vi "Main.vi"() -> ()   [LabVIEW 2024]
doc: "This template is for the Queued Message Handler design pattern.\n\nThe Event Handling Loop generates messages based on user interface actions.\n\nThe Message Handling Loop processes messages generated by the Event Handling Loop, or by other messages. The messages are string values, so new messages can be added easily to the Message Cases case structure in the Message Handling Loop. Each message cluster can also provide an optional value for Message Data, which is a variant that can be converted to whatever message-specific data is required."
uses:
  controls/UI Data.ctl
  <vilib>/Utility/miscctls.llb/LVPointTypeDef.ctl
  <vilib>/Utility/miscctls.llb/LVRectTypeDef.ctl
  support/Message Queue/Enqueue Message (Single).vi
  <vilib>/Instr/_visa.llb/VISA Configure Serial Port (Serial Instr).vi
  support/Message Queue/Message Queue.lvlib
  support/User Event - Stop/User Event - Stop.lvlib
panel:
  in  "Btn-Minimize":bool
  in  "Btn-Close":bool
  in  "Tab ROV":T1(tab)
  in  "Serial-Baudaje":u16(ring) items=["9600"=9600, "19200"=19200, "38400"=38400, "57600"=57600, "115200"=65535]
  in  "Serial-Port":refnum<visa-resource-name>
  in  "Btn-Conectar":bool
  in  "Btn-Desconectar":bool
  out "Serial-State":bool
  out "Numeric 11":dbl
  out "Numeric 10":dbl
  out "Numeric 9":dbl
  out "Numeric 8":dbl
  out "Numeric 7":dbl
  out "Numeric 6":dbl
  out "Numeric 5":dbl
  out "Numeric 4":dbl
  out "Numeric 3":dbl
  out "Numeric 2":dbl
  out "Numeric":dbl
  out "Tecla-S":bool
  out "Tecla-Q":bool
  out "Tecla-E":bool
  out "Tecla-D":bool
  out "Tecla-A":bool
  out "Tecla-W":bool
  in  "Menu4-Propulsores":bool
  in  "Menu3-Inclinacion":bool
  in  "Menu2-Movimientos":bool
  in  "Menu1-Configuracion":bool
  # "Conexión Serial"
  # "Puerto"
  # "Baudaje"
  # "Estado:"
  # "Subir"
  # "Bajar"
  # "Avanzar"
  # "Girar Izquierda"
  # "Retroceder"
  # "Girar Derecha"
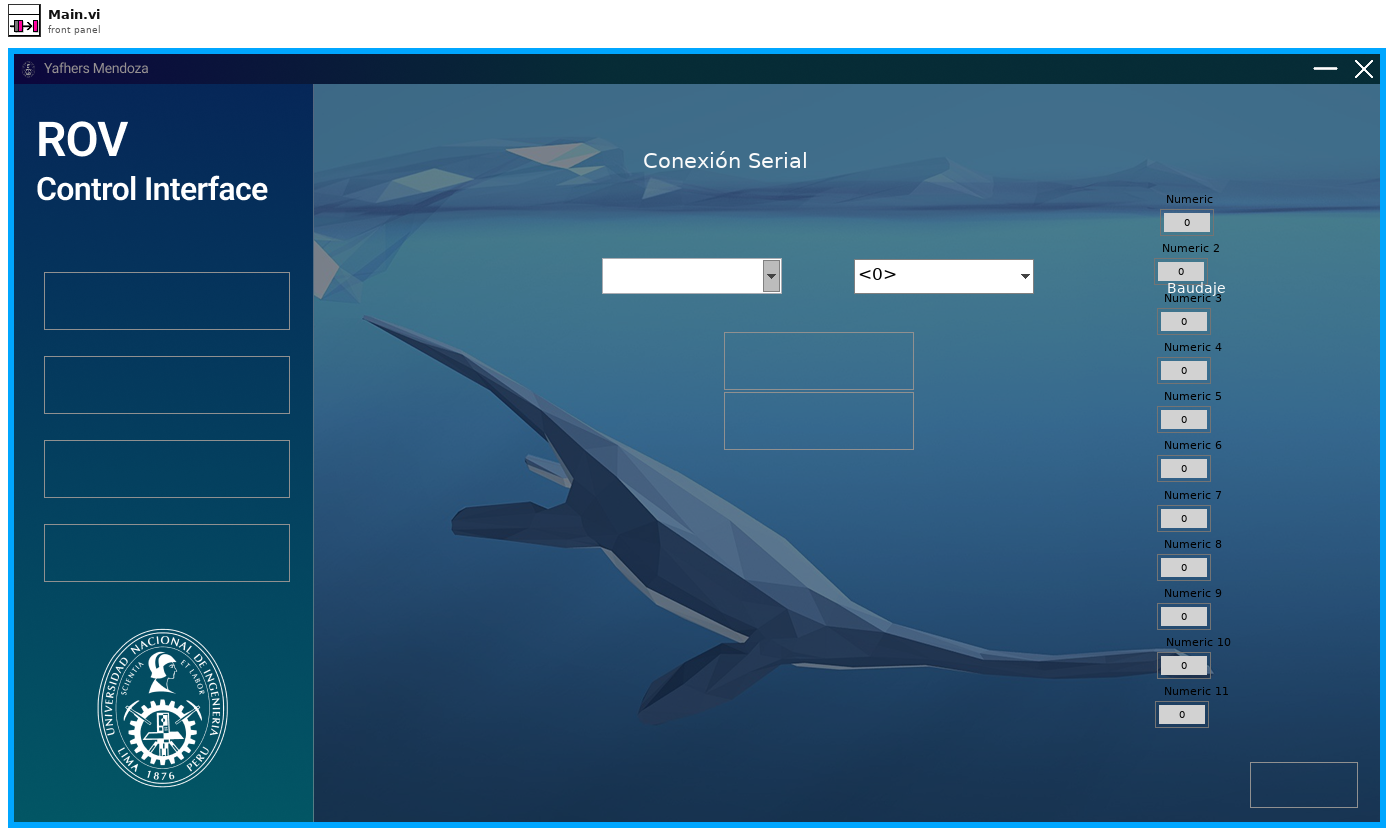
[diagram p1: front panel]
types:
  T1 = enum32{" Tab-Configuracion", "Tab-Movimientos", "Tab-Inclinación", "Tab-Propulsores"}
  T2 = typedef "UI Data.ctl" = cluster{"Data":cluster{"Counter":dbl, "Yaw":dbl, "Pitch":dbl, "Roll":dbl, "Yaw_Desired":dbl, "Pitch_Desired":dbl, "Roll_Desired":dbl, "Motor_Yaw_L":dbl, "Motor_Yaw_R":dbl, "Motor_Pitch_B":dbl, "Motor_Pitch_T":dbl, "Command_Move":dbl}, "Serial":cluster{"Estado":bool, "Puerto":refnum<visa-resource-name>, "Buffer":string}}
  T3 = typedef "Message Queue.lvlib/All Message Queues.ctl" = cluster{"MHL":refnum<queue>, "Loop Serial":refnum<queue>}
  T4 = enum8{"Enabled", "Disabled", "Disabled and Grayed Out"}
  T5 = typedef "LVRectTypeDef.ctl" = cluster{"Left":i16, "Top":i16, "Right":i16, "Bottom":i16}
  T6 = typedef "LVPointTypeDef.ctl" = cluster{"Horizontal":i16, "Vertical":i16}
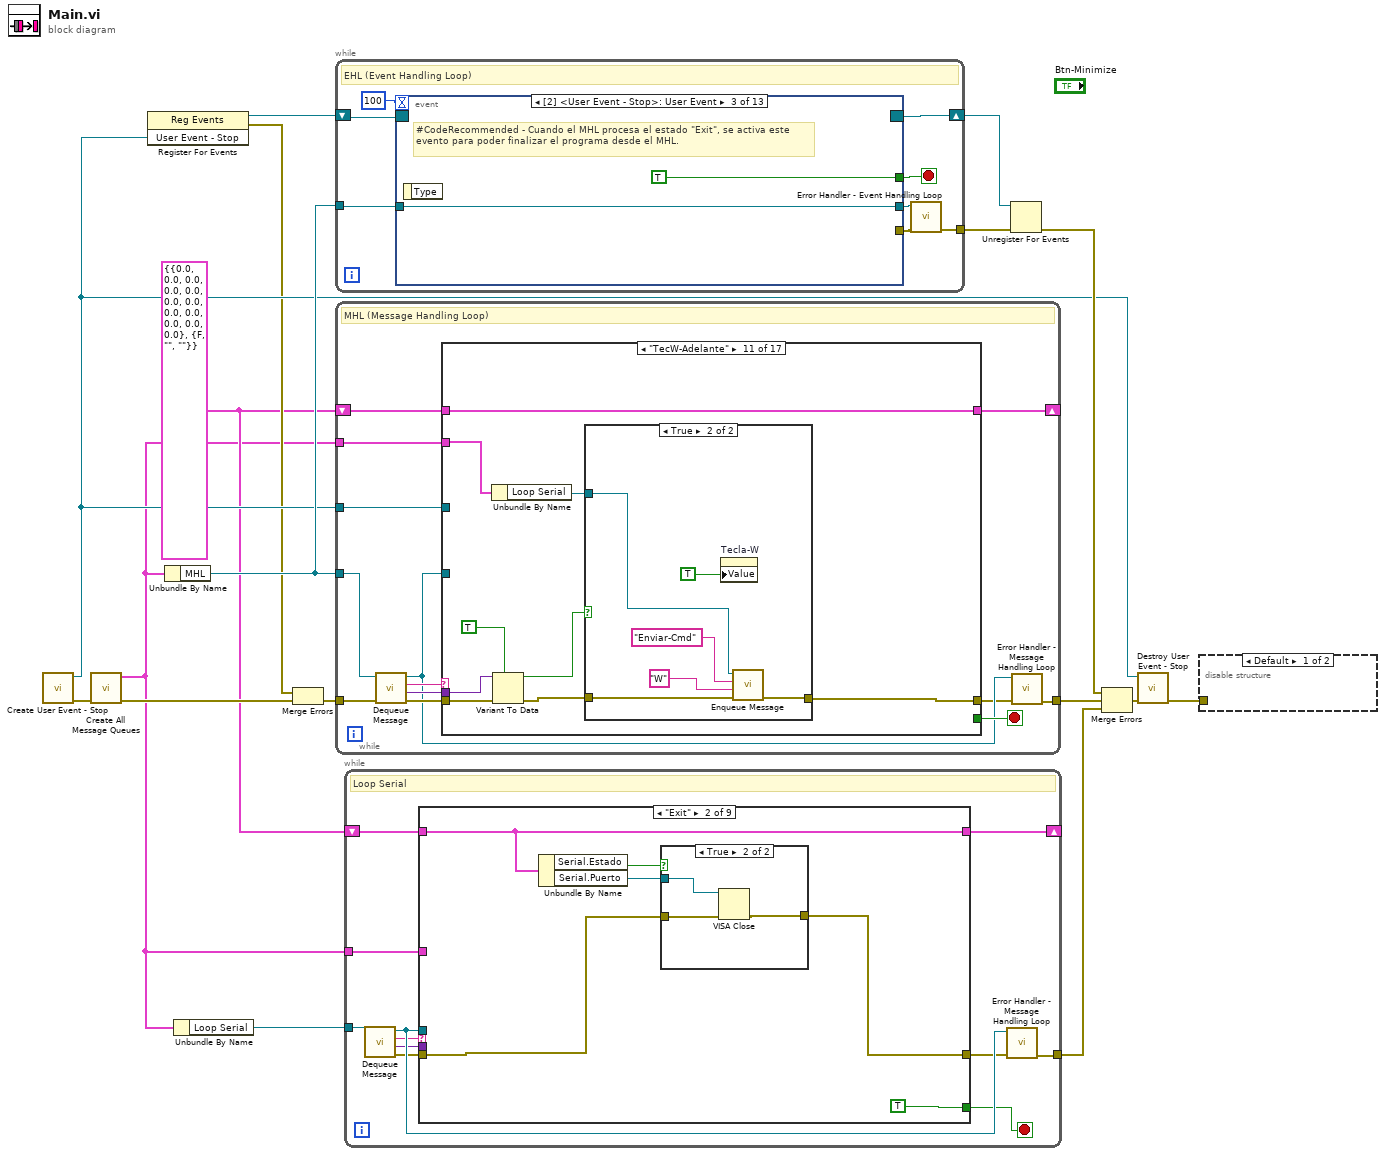
[diagram p0: block diagram]
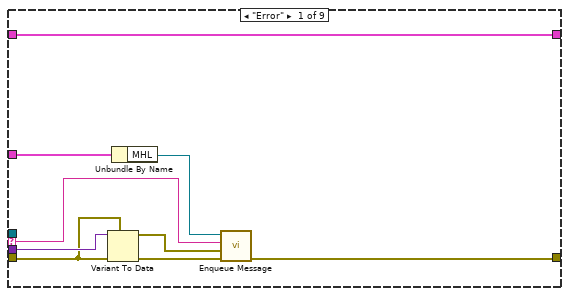
[diagram p2: hidden frame]
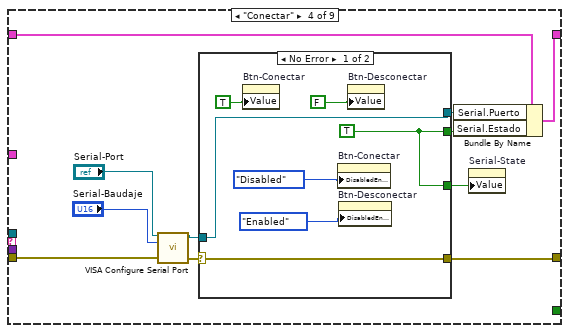
[diagram p5: hidden frame]
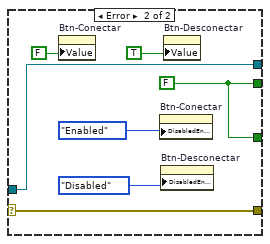
[diagram p6: hidden frame]
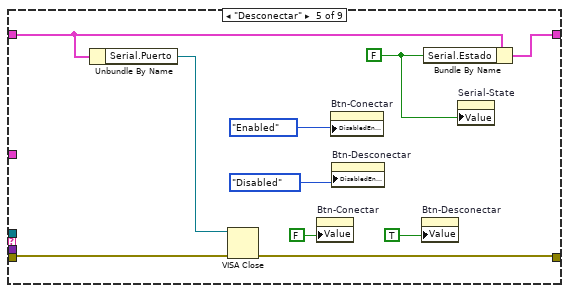
[diagram p7: hidden frame]
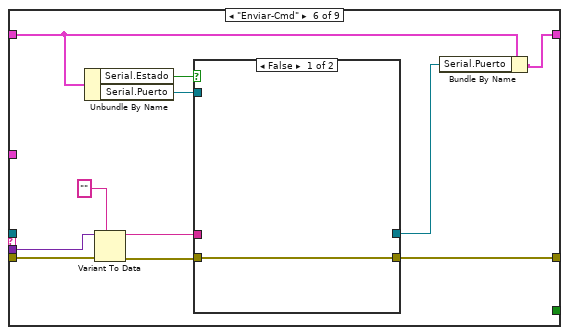
[diagram p8: hidden frame]
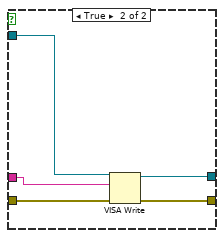
[diagram p9: hidden frame]
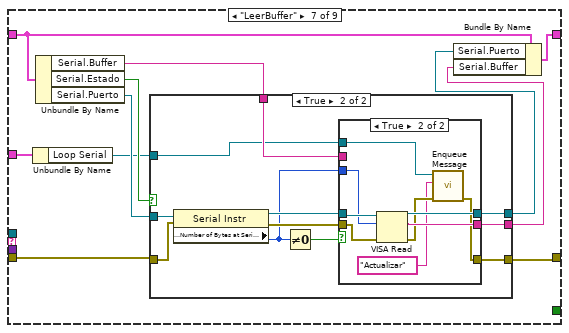
[diagram p10: hidden frame]
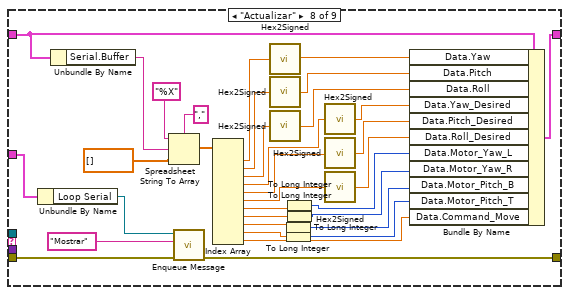
[diagram p13: hidden frame]
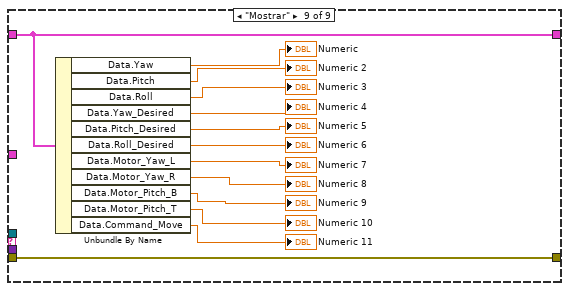
[diagram p14: hidden frame]
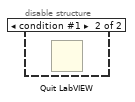
[diagram p15: hidden frame]
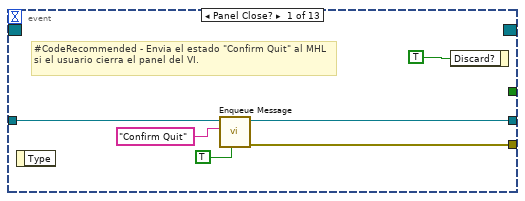
[diagram p16: hidden frame]
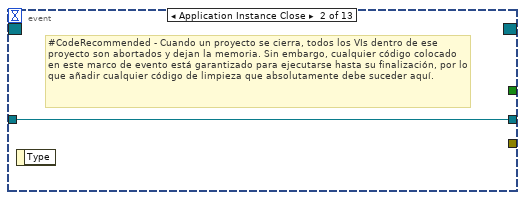
[diagram p17: hidden frame]
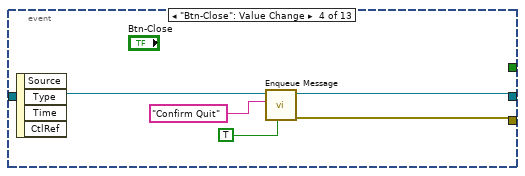
[diagram p18: hidden frame]
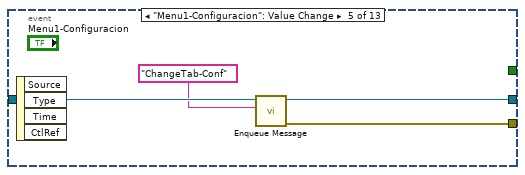
[diagram p19: hidden frame]
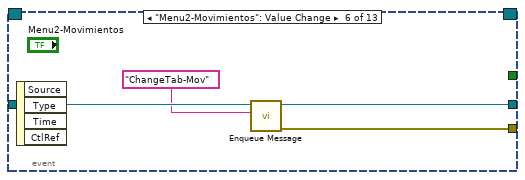
[diagram p20: hidden frame]
diagram:
  w4 = T2 {"Data"={"Counter"=0.0, "Yaw"=0.0, "Pitch"=0.0, "Roll"=0.0, "Yaw_Desired"=0.0, "Pitch_Desired"=0.0, "Roll_Desired"=0.0, "Motor_Yaw_L"=0.0, "Motor_Yaw_R"=0.0, "Motor_Pitch_B"=0.0, "Motor_Pitch_T"=0.0, "Command_Move"=0.0}, "Serial"={"Estado"=FALSE, "Puerto"="", "Buffer"=""}} ("Data Cluster")
  n1 = call "Create User Event - Stop.vi"() -> ("error out"=w14:errorcluster, "User Event - Stop"=w7:refnum<user-event>)  [unwired: 10 in]
  n2 = call "Create All Message Queues.vi"("error in (no error)"=w14) -> ("error out"=w17:errorcluster, "Message Queues out"=w2:T3)  [unwired: 9 in]
  n3 = register-events(w7) -> (reference out=w8:refnum<event-registration>, error out=w5:errorcluster)  [unwired: 2 in]
  n4 = Unbundle By Name(w2) -> ("MHL"=w15:refnum<queue>)
  n5 = Unbundle By Name(w2) -> ("Loop Serial"=w3:refnum<queue>)
  n6 = Merge Errors(w5, w17) -> (w6:errorcluster)
  n7 = while {
    tunnel: w15 -> [w25]
    shift-right: [w23] -> w11
    shift-left: w8 -> [w24]
    tunnel: [w19] -> w9
    stop <- w21 stop-if-true
    # "EHL (Event Handling Loop)"
    n8 = event shown="[2] <User Event - Stop>: User Event" {
      selector: w24 -> [_ _ _ _ _ _ _ _ _ _ _ _ _]
      dyn-events: [_ _ _ _ _ _ _ _ _ _ _ _ _] -> w23
      timeout: 100 -> [_ _ _ _ _ _ _ _ _ _ _ _ _]
      tunnel: [_ _ TRUE ("Discard?") _ _ _ _ _ _ _ _ _ _] -> w21
      tunnel: w25 -> [w30 w32 w34 w37 w43 w47 w51 w55 w59 w63 w67 w102 w137]
      tunnel: [w29 _ _ w38 w42 w46 w50 w54 w58 w61 w66 w101 w135] -> w22
      tunnel: [w28 w32 w34 w39 w41 w45 w49 w53 w57 w62 w65 w100 w136] -> w20
      event Panel Close? {
        # "#CodeRecommended - Envia el estado \"Confirm Quit\" al MHL si el usuario cierra el panel del VI."
        n9 = event-data() -> ()  [unwired: 1 in, 1 out]
        n10 = call-poly "Enqueue Message.vi"("Priority Message? (F)"=TRUE, "Message"="Confirm Quit", "Message Queue"=w30) -> ("error out"=w29:errorcluster, "dup Message Queue"=w28:refnum<queue>)  [unwired: 7 in]
        n11 = event-data("Discard?"=TRUE) -> ()  [unwired: 1 in, 1 out]
      }
      event Application Instance Close {
        # "#CodeRecommended - Cuando un proyecto se cierra, todos los VIs dentro de ese proyecto son abortados y dejan la memoria. Sin embargo, cualquier código colocado en este marco de evento está garantizado para ejecutarse hasta su finalización, por lo que añadir cualquier código de limpieza que absolutamente debe suceder aquí."
        n12 = event-data() -> ()  [unwired: 1 in, 1 out]
      }
      event User Event {
        # "#CodeRecommended - Cuando el MHL procesa el estado \"Exit\", se activa este evento para poder finalizar el programa desde el MHL."
        n13 = event-data() -> ()  [unwired: 1 in, 1 out]
      }
      event "Btn-Close": Value Change {
        n14 = event-data() -> ()  [unwired: 1 in, 4 out]
        n15 = call-poly "Enqueue Message.vi"("Priority Message? (F)"=TRUE, "Message"="Confirm Quit", "Message Queue"=w37) -> ("error out"=w38:errorcluster, "dup Message Queue"=w39:refnum<queue>)  [unwired: 7 in]
      }
      event "Menu1-Configuracion": Value Change {
        n16 = event-data() -> ()  [unwired: 1 in, 4 out]
        n17 = call-poly "Enqueue Message.vi"("Message"="ChangeTab-Conf", "Message Queue"=w43) -> ("error out"=w42:errorcluster, "dup Message Queue"=w41:refnum<queue>)  [unwired: 8 in]
      }
      event "Menu2-Movimientos": Value Change {
        n18 = event-data() -> ()  [unwired: 1 in, 4 out]
        n19 = call-poly "Enqueue Message.vi"("Message"="ChangeTab-Mov", "Message Queue"=w47) -> ("error out"=w46:errorcluster, "dup Message Queue"=w45:refnum<queue>)  [unwired: 8 in]
      }
      event "Menu3-Inclinacion": Value Change {
        n20 = event-data() -> ()  [unwired: 1 in, 4 out]
        n21 = call-poly "Enqueue Message.vi"("Message"="ChangeTab-Inc", "Message Queue"=w51) -> ("error out"=w50:errorcluster, "dup Message Queue"=w49:refnum<queue>)  [unwired: 8 in]
      }
      event "Menu4-Propulsores": Value Change {
        n22 = event-data() -> ()  [unwired: 1 in, 4 out]
        n23 = call-poly "Enqueue Message.vi"("Message"="ChangeTab-Prop", "Message Queue"=w55) -> ("error out"=w54:errorcluster, "dup Message Queue"=w53:refnum<queue>)  [unwired: 8 in]
      }
      event "Btn-Conectar": Value Change {
        n24 = event-data() -> ()  [unwired: 1 in, 4 out]
        n25 = call-poly "Enqueue Message.vi"("Message"="Serial-Conectar", "Message Queue"=w59) -> ("error out"=w58:errorcluster, "dup Message Queue"=w57:refnum<queue>)  [unwired: 8 in]
      }
      event "Btn-Desconectar": Value Change {
        n26 = event-data() -> ()  [unwired: 1 in, 4 out]
        n27 = call-poly "Enqueue Message.vi"("Message"="Serial-Desconectar", "Message Queue"=w63) -> ("error out"=w61:errorcluster, "dup Message Queue"=w62:refnum<queue>)  [unwired: 8 in]
      }
      event Key Down {
        n28 = event-data() -> ("Char"=w64:i16)  [unwired: 1 in, 7 out]
        n29 = case shown="87, 119" w64 {
          tunnel: w67 -> [w68 w73 w78 w83 w88 w93 w98]
          tunnel: [_ w71 w76 w81 w86 w91 w97] -> w66
          tunnel: [w68 w72 w77 w82 w87 w92 w96] -> w65
          frame 0, Default {
          }
          frame 87, 119 {
            # "Tecla W"
            n30 = call-poly "Enqueue Message.vi"("Message Data"=TRUE, "Message"="TecW-Adelante", "Message Queue"=w73) -> ("error out"=w71:errorcluster, "dup Message Queue"=w72:refnum<queue>)  [unwired: 7 in]
          }
          frame 65, 97 {
            # "Tecla A"
            n31 = call-poly "Enqueue Message.vi"("Message Data"=TRUE, "Message"="TecA-GirarIzq", "Message Queue"=w78) -> ("error out"=w76:errorcluster, "dup Message Queue"=w77:refnum<queue>)  [unwired: 7 in]
          }
          frame 68, 100 {
            # "Tecla D"
            n32 = call-poly "Enqueue Message.vi"("Message Data"=TRUE, "Message"="TecD-GirarDer", "Message Queue"=w83) -> ("error out"=w81:errorcluster, "dup Message Queue"=w82:refnum<queue>)  [unwired: 7 in]
          }
          frame 83, 115 {
            # "Tecla S"
            n33 = call-poly "Enqueue Message.vi"("Message Data"=TRUE, "Message"="TecS-Atras", "Message Queue"=w88) -> ("error out"=w86:errorcluster, "dup Message Queue"=w87:refnum<queue>)  [unwired: 7 in]
          }
          frame 81, 113 {
            # "Tecla Q"
            n34 = call-poly "Enqueue Message.vi"("Message Data"=TRUE, "Message"="TecQ-Bajar", "Message Queue"=w93) -> ("error out"=w91:errorcluster, "dup Message Queue"=w92:refnum<queue>)  [unwired: 7 in]
          }
          frame 69, 101 {
            # "Tecla E"
            n35 = call-poly "Enqueue Message.vi"("Message Data"=TRUE, "Message"="TecE-Subir", "Message Queue"=w98) -> ("error out"=w97:errorcluster, "dup Message Queue"=w96:refnum<queue>)  [unwired: 7 in]
          }
        }
      }
      event Key Up {
        n36 = event-data() -> ("ScanCode"=w99:i16)  [unwired: 1 in, 7 out]
        n37 = case shown="0, Default" w99 {
          tunnel: w102 -> [w103 w108 w113 w118 w123 w128 w133]
          tunnel: [_ w106 w111 w116 w121 w126 w132] -> w101
          tunnel: [w103 w107 w112 w117 w122 w127 w131] -> w100
          frame 0, Default {
          }
          frame 17 {
            # "Tecla W"
            n38 = call-poly "Enqueue Message.vi"("Message Data"=FALSE, "Message"="TecW-Adelante", "Message Queue"=w108) -> ("error out"=w106:errorcluster, "dup Message Queue"=w107:refnum<queue>)  [unwired: 7 in]
          }
          frame 30 {
            # "Tecla A"
            n39 = call-poly "Enqueue Message.vi"("Message Data"=FALSE, "Message"="TecA-GirarIzq", "Message Queue"=w113) -> ("error out"=w111:errorcluster, "dup Message Queue"=w112:refnum<queue>)  [unwired: 7 in]
          }
          frame 32 {
            # "Tecla D"
            n40 = call-poly "Enqueue Message.vi"("Message Data"=FALSE, "Message"="TecD-GirarDer", "Message Queue"=w118) -> ("error out"=w116:errorcluster, "dup Message Queue"=w117:refnum<queue>)  [unwired: 7 in]
          }
          frame 31 {
            # "Tecla S"
            n41 = call-poly "Enqueue Message.vi"("Message Data"=FALSE, "Message"="TecS-Atras", "Message Queue"=w123) -> ("error out"=w121:errorcluster, "dup Message Queue"=w122:refnum<queue>)  [unwired: 7 in]
          }
          frame 16 {
            # "Tecla Q"
            n42 = call-poly "Enqueue Message.vi"("Message Data"=FALSE, "Message"="TecQ-Bajar", "Message Queue"=w128) -> ("error out"=w126:errorcluster, "dup Message Queue"=w127:refnum<queue>)  [unwired: 7 in]
          }
          frame 18 {
            # "Tecla E"
            n43 = call-poly "Enqueue Message.vi"("Message Data"=FALSE, "Message"="TecE-Subir", "Message Queue"=w133) -> ("error out"=w132:errorcluster, "dup Message Queue"=w131:refnum<queue>)  [unwired: 7 in]
          }
        }
      }
      event Timeout {
        n44 = event-data() -> ()  [unwired: 1 in, 3 out]
        n45 = call-poly "Enqueue Message.vi"("Message"="Serial-CollectData", "Message Queue"=w137) -> ("error out"=w135:errorcluster, "dup Message Queue"=w136:refnum<queue>)  [unwired: 8 in]
      }
    }
    n46 = call "Error Handler - Event Handling Loop.vi"("error in (no error)"=w22, "Message Queue"=w20) -> ("dup error in"=w19:errorcluster)  [unwired: 8 in, 1 out]
  }
  n47 = while {
    tunnel: w15 -> [w142]
    shift-right: [w149] -> _
    shift-left: w4 -> [w150]
    tunnel: w7 -> [w147]
    tunnel: w6 -> [w146]
    tunnel: [w140] -> w16
    tunnel: w2 -> [w138]
    stop <- w148 stop-if-true
    # "MHL (Message Handling Loop)"
    n48 = call "Dequeue Message.vi"("error in (no error)"=w146, "Message Queue"=w142) -> ("error out"=w145:errorcluster, "Message Data"=w143:variant, "Message"=w144:string, "dup Message Queue"=w141:refnum<queue>)  [unwired: 6 in]
    n49 = case "Message Cases" shown="\"TecW-Adelante\"" w144 {
      tunnel: w141 -> [_ _ w189 _ _ _ _ _ _ _ _ _ _ _ _ _ w375]
      tunnel: w145 -> [w173 w180 w192 w199 w206 w213 w220 w224 w230 w236 w246 w266 w287 w308 w329 w350 w368]
      tunnel: [w173 w174 w190 w199 w206 w213 w220 w223 w227 w235 w240 w262 w282 w304 w325 w346 w371] -> w139
      tunnel: w150 -> [w172 w179 w191 w198 w205 w212 w219 w226 w232 w238 w247 w268 w289 w310 w331 w352 w374]
      tunnel: [w172 w179 w191 w198 w205 w212 w219 w226 w232 w238 w247 w268 w289 w310 w331 w352 w374] -> w149
      tunnel: [_ _ _ _ _ _ _ _ _ _ _ _ _ _ _ _ TRUE] -> w148
      tunnel: w143 -> [_ w178 _ _ _ _ _ _ _ _ w245 w265 w286 w306 w328 w349 w365]
      tunnel: w147 -> [_ _ _ _ _ _ _ _ _ _ _ _ _ _ _ _ w370]
      tunnel: w138 -> [_ _ w186 _ _ _ _ w225 w231 w237 w242 w261 w284 w303 w324 w345 _]
      frame "Initialize", Default {
        w153 = FALSE ("Serial-State")
        # "#CodeRecommended - Estado de Inicialización por defecto."
        # "Initialize - All initialization work should take place in this message, since other loops can potentially enqueue messages that execute immediately after this one."
        n50 = property on="Pane" class="Pane"("Origin"=T6 {"Horizontal"=0, "Vertical"=0}) -> ()  [unwired: 2 in, 2 out]
        n51 = Current VI's Path() -> (path=w169:path)
        n52 = property on="Btn-Conectar" class="Bool (strict)"("DisabledEnum"=T4."Enabled" ("Disabled")) -> ()  [unwired: 2 in, 2 out]
        n53 = property on="Menu3-Inclinacion" class="Bool (strict)"("DisabledEnum"=T4."Disabled" ("Disabled")) -> ()  [unwired: 2 in, 2 out]
        n54 = property on="Menu4-Propulsores" class="Bool (strict)"("DisabledEnum"=T4."Disabled" ("Disabled")) -> ()  [unwired: 2 in, 2 out]
        n55 = property on="Btn-Desconectar" class="Bool (strict)"("DisabledEnum"=T4."Enabled" ("Disabled")) -> ()  [unwired: 2 in, 2 out]
        n56 = Open VI Reference(vi path=w169) -> (vi reference=w168:refnum<vi>, error out=w167:errorcluster)  [unwired: 5 in]
        n57 = property on="Tab ROV" class="TabCtl (strict)"("Value"=T1." Tab-Configuracion" ("Tab ROV")) -> ()  [unwired: 2 in, 2 out]
        n58 = property class="VI"(reference=w168, error in=w167, "Front Panel.PanelBounds"=T5 {"Left"=300, "Top"=120, "Right"=1366, "Bottom"=768} ("Front Panel Window:Panel Bounds")) -> (reference out=w166:refnum<vi>, error out=w165:errorcluster)
        n59 = property on="Menu4-Propulsores" class="Bool (strict)"("Value"=FALSE) -> ()  [unwired: 2 in, 2 out]
        n60 = property on="Menu2-Movimientos" class="Bool (strict)"("Value"=FALSE) -> ()  [unwired: 2 in, 2 out]
        n61 = property on="Menu1-Configuracion" class="Bool (strict)"("Value"=TRUE) -> ()  [unwired: 2 in, 2 out]
        n62 = property on="Menu3-Inclinacion" class="Bool (strict)"("Value"=FALSE) -> ()  [unwired: 2 in, 2 out]
        n63 = property on="Btn-Conectar" class="Bool (strict)"("Value"=FALSE) -> ()  [unwired: 2 in, 2 out]
        n64 = Close Reference(reference=w166, error in (no error)=w165) -> ()  [unwired: 1 out]
        n65 = property on="Btn-Desconectar" class="Bool (strict)"("Value"=FALSE) -> ()  [unwired: 2 in, 2 out]
        n66 = property on="Serial-State" class="Bool"("Value"=FALSE) -> ()  [unwired: 2 in, 2 out]
        "Serial-State" <- FALSE ("Serial-State")
        "Tecla-W" <- w153
        "Tecla-D" <- w153
        "Tecla-A" <- w153
        "Tecla-S" <- w153
        "Tecla-Q" <- w153
        "Tecla-E" <- w153
      }
      frame "Error" {
        # "#CodeRecommended - Muestra un diálogo de error. Este mensaje es enviado por los VIs «Error Handler» al final de otros bucles en esta aplicación.."
        # "Error - Display an error dialog. This message is sent by the \"Error Handler\" VIs at the end of other loops in this application."
        n67 = Variant To Data(error in=w180, type=errorcluster {"status"=FALSE, "code"=0, "source"=""} ("error constant"), Variant=w178) -> (data=w176:errorcluster, error out=w175:errorcluster)
        n68 = call <vilib>:"Simple Error Handler.vi"("error in (no error)"=w176) -> ()  [unwired: 4 in, 5 out]
        n69 = Merge Errors(w175) -> (w174:errorcluster)
      }
      frame "Confirm Quit" {
        # "#CodeRecommended - Estado para confirmar que el usuario desea salir de la aplicación, asegurese de cerrar todos sus bucles en este estado."
        # "Confirm Quit - Message that can confirm whether or not the user wants to exit the application."
        n70 = Unbundle By Name(w186) -> ("Loop Serial"=w184:refnum<queue>)
        n71 = call-poly "Enqueue Message.vi"("Priority Message? (F)"=TRUE, "error in (no error)"=w192, "Message"="Exit", "Message Queue"=w189) -> ("error out"=w185:errorcluster)  [unwired: 6 in, 1 out]
        n72 = call-poly "Enqueue Message.vi"("Priority Message? (F)"=TRUE, "error in (no error)"=w185, "Message"="Exit", "Message Queue"=w184) -> ("error out"=w181:errorcluster)  [unwired: 6 in, 1 out]
        n73 = Merge Errors(w181) -> (w190:errorcluster)
      }
      frame "ChangeTab-Conf" {
        n74 = property on="Menu2-Movimientos" class="Bool (strict)"("Value"=FALSE) -> ()  [unwired: 2 in, 2 out]
        n75 = property on="Menu1-Configuracion" class="Bool (strict)"("Value"=TRUE) -> ()  [unwired: 2 in, 2 out]
        n76 = property on="Menu4-Propulsores" class="Bool (strict)"("Value"=FALSE) -> ()  [unwired: 2 in, 2 out]
        n77 = property on="Menu3-Inclinacion" class="Bool (strict)"("Value"=FALSE) -> ()  [unwired: 2 in, 2 out]
        n78 = property on="Tab ROV" class="TabCtl (strict)"("Value"=T1." Tab-Configuracion" ("Tab ROV")) -> ()  [unwired: 2 in, 2 out]
      }
      frame "ChangeTab-Mov" {
        n79 = property on="Menu2-Movimientos" class="Bool (strict)"("Value"=TRUE) -> ()  [unwired: 2 in, 2 out]
        n80 = property on="Menu1-Configuracion" class="Bool (strict)"("Value"=FALSE) -> ()  [unwired: 2 in, 2 out]
        n81 = property on="Menu4-Propulsores" class="Bool (strict)"("Value"=FALSE) -> ()  [unwired: 2 in, 2 out]
        n82 = property on="Menu3-Inclinacion" class="Bool (strict)"("Value"=FALSE) -> ()  [unwired: 2 in, 2 out]
        n83 = property on="Tab ROV" class="TabCtl (strict)"("Value"=T1."Tab-Movimientos" ("Tab ROV")) -> ()  [unwired: 2 in, 2 out]
      }
      frame "ChangeTab-Inc" {
        n84 = property on="Menu2-Movimientos" class="Bool (strict)"("Value"=FALSE) -> ()  [unwired: 2 in, 2 out]
        n85 = property on="Menu1-Configuracion" class="Bool (strict)"("Value"=FALSE) -> ()  [unwired: 2 in, 2 out]
        n86 = property on="Menu4-Propulsores" class="Bool (strict)"("Value"=FALSE) -> ()  [unwired: 2 in, 2 out]
        n87 = property on="Menu3-Inclinacion" class="Bool (strict)"("Value"=TRUE) -> ()  [unwired: 2 in, 2 out]
        n88 = property on="Tab ROV" class="TabCtl (strict)"("Value"=T1."Tab-Inclinación" ("Tab ROV")) -> ()  [unwired: 2 in, 2 out]
      }
      frame "ChangeTab-Prop" {
        n89 = property on="Menu2-Movimientos" class="Bool (strict)"("Value"=FALSE) -> ()  [unwired: 2 in, 2 out]
        n90 = property on="Menu1-Configuracion" class="Bool (strict)"("Value"=FALSE) -> ()  [unwired: 2 in, 2 out]
        n91 = property on="Menu4-Propulsores" class="Bool (strict)"("Value"=TRUE) -> ()  [unwired: 2 in, 2 out]
        n92 = property on="Menu3-Inclinacion" class="Bool (strict)"("Value"=FALSE) -> ()  [unwired: 2 in, 2 out]
        n93 = property on="Tab ROV" class="TabCtl (strict)"("Value"=T1."Tab-Propulsores" ("Tab ROV")) -> ()  [unwired: 2 in, 2 out]
      }
      frame "Serial-Conectar" {
        n94 = Unbundle By Name(w225) -> ("Loop Serial"=w222:refnum<queue>)
        n95 = call-poly "Enqueue Message.vi"("error in (no error)"=w224, "Message"="Conectar", "Message Queue"=w222) -> ("error out"=w223:errorcluster)  [unwired: 7 in, 1 out]
      }
      frame "Serial-Desconectar" {
        n96 = Unbundle By Name(w231) -> ("Loop Serial"=w229:refnum<queue>)
        n97 = call-poly "Enqueue Message.vi"("error in (no error)"=w230, "Message"="Desconectar", "Message Queue"=w229) -> ("error out"=w227:errorcluster)  [unwired: 7 in, 1 out]
      }
      frame "Serial-CollectData" {
        n98 = Unbundle By Name(w237) -> ("Loop Serial"=w234:refnum<queue>)
        n99 = call-poly "Enqueue Message.vi"("error in (no error)"=w236, "Message"="LeerBuffer", "Message Queue"=w234) -> ("error out"=w235:errorcluster)  [unwired: 7 in, 1 out]
      }
      frame "TecW-Adelante" {
        n100 = Unbundle By Name(w242) -> ("Loop Serial"=w239:refnum<queue>)
        n101 = Variant To Data(error in=w246, type=TRUE, Variant=w245) -> (data=w243:bool, error out=w241:errorcluster)
        n102 = case shown="True" w243 {
          tunnel: w241 -> [w252 w256]
          tunnel: [w251 w255] -> w240
          tunnel: w239 -> [w249 w254]
          frame False {
            n103 = property on="Tecla-W" class="Bool"("Value"=FALSE ("Tecla-W")) -> ()  [unwired: 2 in, 2 out]
            n104 = call-poly "Enqueue Message.vi"("error in (no error)"=w252, "Message Data"="w", "Message"="Enviar-Cmd", "Message Queue"=w249) -> ("error out"=w251:errorcluster)  [unwired: 6 in, 1 out]
          }
          frame True {
            n105 = property on="Tecla-W" class="Bool"("Value"=TRUE ("Tecla-W")) -> ()  [unwired: 2 in, 2 out]
            n106 = call-poly "Enqueue Message.vi"("error in (no error)"=w256, "Message Data"="W", "Message"="Enviar-Cmd", "Message Queue"=w254) -> ("error out"=w255:errorcluster)  [unwired: 6 in, 1 out]
          }
        }
      }
      frame "TecD-GirarDer" {
        n107 = Unbundle By Name(w261) -> ("Loop Serial"=w260:refnum<queue>)
        n108 = Variant To Data(error in=w266, type=TRUE, Variant=w265) -> (data=w264:bool, error out=w263:errorcluster)
        n109 = case shown="True" w264 {
          tunnel: w263 -> [w271 w277]
          tunnel: [w270 w276] -> w262
          tunnel: w260 -> [w269 w275]
          frame False {
            n110 = property on="Tecla-D" class="Bool"("Value"=FALSE ("Tecla-D")) -> ()  [unwired: 2 in, 2 out]
            n111 = call-poly "Enqueue Message.vi"("error in (no error)"=w271, "Message Data"="d", "Message"="Enviar-Cmd", "Message Queue"=w269) -> ("error out"=w270:errorcluster)  [unwired: 6 in, 1 out]
          }
          frame True {
            n112 = property on="Tecla-D" class="Bool"("Value"=TRUE ("Tecla-D")) -> ()  [unwired: 2 in, 2 out]
            n113 = call-poly "Enqueue Message.vi"("error in (no error)"=w277, "Message Data"="D", "Message"="Enviar-Cmd", "Message Queue"=w275) -> ("error out"=w276:errorcluster)  [unwired: 6 in, 1 out]
          }
        }
      }
      frame "TecA-GirarIzq" {
        n114 = Unbundle By Name(w284) -> ("Loop Serial"=w281:refnum<queue>)
        n115 = Variant To Data(error in=w287, type=TRUE, Variant=w286) -> (data=w285:bool, error out=w283:errorcluster)
        n116 = case shown="True" w285 {
          tunnel: w283 -> [w292 w298]
          tunnel: [w291 w297] -> w282
          tunnel: w281 -> [w290 w296]
          frame False {
            n117 = property on="Tecla-A" class="Bool"("Value"=FALSE ("Tecla-A")) -> ()  [unwired: 2 in, 2 out]
            n118 = call-poly "Enqueue Message.vi"("error in (no error)"=w292, "Message Data"="a", "Message"="Enviar-Cmd", "Message Queue"=w290) -> ("error out"=w291:errorcluster)  [unwired: 6 in, 1 out]
          }
          frame True {
            n119 = property on="Tecla-A" class="Bool"("Value"=TRUE ("Tecla-A")) -> ()  [unwired: 2 in, 2 out]
            n120 = call-poly "Enqueue Message.vi"("error in (no error)"=w298, "Message Data"="A", "Message"="Enviar-Cmd", "Message Queue"=w296) -> ("error out"=w297:errorcluster)  [unwired: 6 in, 1 out]
          }
        }
      }
      frame "TecS-Atras" {
        n121 = Unbundle By Name(w303) -> ("Loop Serial"=w302:refnum<queue>)
        n122 = Variant To Data(error in=w308, type=TRUE, Variant=w306) -> (data=w307:bool, error out=w305:errorcluster)
        n123 = case shown="False" w307 {
          tunnel: w305 -> [w313 w319]
          tunnel: [w312 w318] -> w304
          tunnel: w302 -> [w311 w317]
          frame False {
            n124 = property on="Tecla-S" class="Bool"("Value"=FALSE ("Tecla-S")) -> ()  [unwired: 2 in, 2 out]
            n125 = call-poly "Enqueue Message.vi"("error in (no error)"=w313, "Message Data"="s", "Message"="Enviar-Cmd", "Message Queue"=w311) -> ("error out"=w312:errorcluster)  [unwired: 6 in, 1 out]
          }
          frame True {
            n126 = property on="Tecla-S" class="Bool"("Value"=TRUE ("Tecla-S")) -> ()  [unwired: 2 in, 2 out]
            n127 = call-poly "Enqueue Message.vi"("error in (no error)"=w319, "Message Data"="S", "Message"="Enviar-Cmd", "Message Queue"=w317) -> ("error out"=w318:errorcluster)  [unwired: 6 in, 1 out]
          }
        }
      }
      frame "TecQ-Bajar" {
        n128 = Unbundle By Name(w324) -> ("Loop Serial"=w323:refnum<queue>)
        n129 = Variant To Data(error in=w329, type=TRUE, Variant=w328) -> (data=w327:bool, error out=w326:errorcluster)
        n130 = case shown="False" w327 {
          tunnel: w326 -> [w334 w340]
          tunnel: [w333 w339] -> w325
          tunnel: w323 -> [w332 w338]
          frame False {
            n131 = property on="Tecla-Q" class="Bool"("Value"=FALSE ("Tecla-Q")) -> ()  [unwired: 2 in, 2 out]
            n132 = call-poly "Enqueue Message.vi"("error in (no error)"=w334, "Message Data"="q", "Message"="Enviar-Cmd", "Message Queue"=w332) -> ("error out"=w333:errorcluster)  [unwired: 6 in, 1 out]
          }
          frame True {
            n133 = property on="Tecla-Q" class="Bool"("Value"=TRUE ("Tecla-Q")) -> ()  [unwired: 2 in, 2 out]
            n134 = call-poly "Enqueue Message.vi"("error in (no error)"=w340, "Message Data"="Q", "Message"="Enviar-Cmd", "Message Queue"=w338) -> ("error out"=w339:errorcluster)  [unwired: 6 in, 1 out]
          }
        }
      }
      frame "TecE-Subir" {
        n135 = Unbundle By Name(w345) -> ("Loop Serial"=w344:refnum<queue>)
        n136 = Variant To Data(error in=w350, type=TRUE, Variant=w349) -> (data=w348:bool, error out=w347:errorcluster)
        n137 = case shown="False" w348 {
          tunnel: w347 -> [w355 w361]
          tunnel: [w354 w360] -> w346
          tunnel: w344 -> [w353 w359]
          frame False {
            n138 = property on="Tecla-E" class="Bool"("Value"=FALSE ("Tecla-E")) -> ()  [unwired: 2 in, 2 out]
            n139 = call-poly "Enqueue Message.vi"("error in (no error)"=w355, "Message Data"="e", "Message"="Enviar-Cmd", "Message Queue"=w353) -> ("error out"=w354:errorcluster)  [unwired: 6 in, 1 out]
          }
          frame True {
            n140 = property on="Tecla-E" class="Bool"("Value"=TRUE ("Tecla-E")) -> ()  [unwired: 2 in, 2 out]
            n141 = call-poly "Enqueue Message.vi"("error in (no error)"=w361, "Message Data"="E", "Message"="Enviar-Cmd", "Message Queue"=w359) -> ("error out"=w360:errorcluster)  [unwired: 6 in, 1 out]
          }
        }
      }
      frame "Exit" {
        # "#CodeRecommended - Añada aquí cualquier código de limpieza necesario. Tenga en cuenta que si 'EXIT' fue llamado como resultado de un error, se mostrará un diálogo de error. Añada también aquí cualquier gestión de error personalizada para una condición 'Salir'."
        # "Exit - Exit the application."
        n142 = Variant To Data(type=errorcluster {"status"=FALSE, "code"=0, "source"=""} ("error constant"), Variant=w365) -> (data=w366:errorcluster)  [unwired: 1 in, 1 out]
        n143 = call <vilib>:"Simple Error Handler.vi"("error in (no error)"=w366) -> ()  [unwired: 4 in, 5 out]
        n144 = call "Fire User Event - Stop.vi"("User Event - Stop"=w370) -> ("error out"=w369:errorcluster)  [unwired: 10 in]
        n145 = Release Queue(queue=w375, error in (no error)=w368) -> (error out=w372:errorcluster)  [unwired: 1 in, 2 out]
        n146 = Merge Errors(w369, w372) -> (w371:errorcluster)
      }
    }
    n147 = call "Error Handler - Message Handling Loop.vi"("error in (no error)"=w139, "Message Queue"=w141) -> ("dup error in"=w140:errorcluster)  [unwired: 8 in, 1 out]
  }
  n148 = while {
    shift-right: [w379] -> _
    shift-left: w4 -> [w378]
    tunnel: [w381] -> w1
    tunnel: w3 -> [w380]
    tunnel: w2 -> [w377]
    stop <- w376 stop-if-true
    # "Loop Serial"
    n149 = call "Dequeue Message.vi"("Message Queue"=w380) -> ("error out"=w384:errorcluster, "Message Data"=w383:variant, "Message"=w385:string, "dup Message Queue"=w386:refnum<queue>)  [unwired: 7 in]
    n150 = case shown="\"Exit\"" w385 {
      selector: w385 -> [w389 _ _ _ _ _ _ _ _]
      tunnel: w386 -> [_ _ _ _ _ _ _ _ _]
      tunnel: w384 -> [w393 w397 w407 w418 w442 w447 w468 w521 w541]
      tunnel: w383 -> [w394 _ _ _ _ w445 _ _ _]
      tunnel: [w387 w396 w407 w411 w440 w452 w469 w520 w541] -> w382
      tunnel: [w395 w400 w406 w414 w438 w449 w465 w529 w542] -> w379
      tunnel: w378 -> [w395 w400 w406 w413 w439 w450 w466 w528 w542]
      tunnel: w377 -> [w392 _ _ _ _ _ w461 w519 _]
      tunnel: [_ TRUE _ _ _ _ _ _ _] -> w376
      frame "Error" {
        n151 = Variant To Data(error in=w393, type=w393, Variant=w394) -> (data=w388:errorcluster, error out=w391:errorcluster)
        n152 = Unbundle By Name(w392) -> ("MHL"=w390:refnum<queue>)
        n153 = call-poly "Enqueue Message.vi"("error in (no error)"=w391, "Message Data"=w388, "Message"=w389, "Message Queue"=w390) -> ("error out"=w387:errorcluster)  [unwired: 6 in, 1 out]
      }
      frame "Exit" {
        n154 = Unbundle By Name(w400) -> ("Serial.Estado"=w399:bool, "Serial.Puerto"=w398:refnum<visa-resource-name>)
        n155 = case shown="True" w399 {
          tunnel: w398 -> [_ w405]
          tunnel: w397 -> [w402 w404]
          tunnel: [w402 w403] -> w396
          frame False {
          }
          frame True {
            n156 = VISA Close(VISA resource name=w405, error in (no error)=w404) -> (error out=w403:errorcluster)
          }
        }
      }
      frame "Initialize", Default {
      }
      frame "Conectar" {
        n157 = call-poly "VISA Configure Serial Port"("VISA resource name"="Serial-Port", "baud rate (9600)"="Serial-Baudaje", "error in (no error)"=w418) -> ("VISA resource name out"=w412:refnum<visa-resource-name>, "error out"=w415:errorcluster)  [unwired: 11 in]
        n158 = case shown="No Error" w415 {
          selector: w415 -> [w424 w431]
          tunnel: [w425 w432] -> w410
          tunnel: w412 -> [w425 w432]
          tunnel: [w424 w431] -> w411
          tunnel: [w421 w428] -> w409
          tunnel: [w421 w428] -> w408
          frame No Error {
            w421 = TRUE
            n159 = property on="Btn-Conectar" class="Bool (strict)"("Value"=TRUE ("Btn-Conectar")) -> ()  [unwired: 2 in, 2 out]
            n160 = property on="Btn-Conectar" class="Bool (strict)"("DisabledEnum"=T4."Disabled" ("Disabled")) -> ()  [unwired: 2 in, 2 out]
            n161 = property on="Btn-Desconectar" class="Bool (strict)"("DisabledEnum"=T4."Enabled" ("Disabled")) -> ()  [unwired: 2 in, 2 out]
            n162 = property on="Btn-Desconectar" class="Bool (strict)"("Value"=FALSE ("Btn-Desconectar")) -> ()  [unwired: 2 in, 2 out]
          }
          frame Error {
            w428 = FALSE
            n163 = property on="Btn-Conectar" class="Bool (strict)"("Value"=FALSE ("Btn-Conectar")) -> ()  [unwired: 2 in, 2 out]
            n164 = property on="Btn-Conectar" class="Bool (strict)"("DisabledEnum"=T4."Enabled" ("Disabled")) -> ()  [unwired: 2 in, 2 out]
            n165 = property on="Btn-Desconectar" class="Bool (strict)"("DisabledEnum"=T4."Disabled" ("Disabled")) -> ()  [unwired: 2 in, 2 out]
            n166 = property on="Btn-Desconectar" class="Bool (strict)"("Value"=TRUE ("Btn-Desconectar")) -> ()  [unwired: 2 in, 2 out]
          }
        }
        n167 = Bundle By Name(cluster=w413, "Serial.Puerto"=w410, "Serial.Estado"=w409) -> (w414:T2)
        n168 = property on="Serial-State" class="Bool"("Value"=w408) -> ()  [unwired: 2 in, 2 out]
      }
      frame "Desconectar" {
        w437 = FALSE ("Serial.Estado")
        n169 = Unbundle By Name(w439) -> ("Serial.Puerto"=w441:refnum<visa-resource-name>)
        n170 = VISA Close(VISA resource name=w441, error in (no error)=w442) -> (error out=w440:errorcluster)
        n171 = property on="Btn-Conectar" class="Bool (strict)"("Value"=FALSE ("Btn-Conectar")) -> ()  [unwired: 2 in, 2 out]
        n172 = property on="Btn-Conectar" class="Bool (strict)"("DisabledEnum"=T4."Enabled" ("Disabled")) -> ()  [unwired: 2 in, 2 out]
        n173 = property on="Btn-Desconectar" class="Bool (strict)"("DisabledEnum"=T4."Disabled" ("Disabled")) -> ()  [unwired: 2 in, 2 out]
        n174 = property on="Btn-Desconectar" class="Bool (strict)"("Value"=TRUE ("Btn-Desconectar")) -> ()  [unwired: 2 in, 2 out]
        n175 = Bundle By Name(cluster=w439, "Serial.Estado"=w437) -> (w438:T2)
        n176 = property on="Serial-State" class="Bool"("Value"=w437) -> ()  [unwired: 2 in, 2 out]
      }
      frame "Enviar-Cmd" {
        n177 = Unbundle By Name(w450) -> ("Serial.Estado"=w453:bool, "Serial.Puerto"=w451:refnum<visa-resource-name>)
        n178 = Variant To Data(error in=w447, type="", Variant=w445) -> (data=w443:string, error out=w446:errorcluster)
        n179 = case shown="False" w453 {
          tunnel: w446 -> [w454 w459]
          tunnel: [w454 w458] -> w452
          tunnel: w451 -> [_ w457]
          tunnel: [_ w456] -> w448
          tunnel: w443 -> [_ w455]
          frame False {
          }
          frame True {
            n180 = VISA Write(VISA resource name=w457, write buffer=w455, error in (no error)=w459) -> (VISA resource name out=w456:refnum<visa-resource-name>, error out=w458:errorcluster)  [unwired: 1 out]
          }
        }
        n181 = Bundle By Name(cluster=w450, "Serial.Puerto"=w448) -> (w449:T2)
      }
      frame "LeerBuffer" {
        n182 = Unbundle By Name(w461) -> ("Loop Serial"=w460:refnum<queue>)
        n183 = Unbundle By Name(w466) -> ("Serial.Buffer"=w462:string, "Serial.Estado"=w470:bool, "Serial.Puerto"=w467:refnum<visa-resource-name>)
        n184 = case shown="True" w470 {
          tunnel: [w473 w479] -> w469
          tunnel: w468 -> [w473 w483]
          tunnel: w467 -> [w472 w484]
          tunnel: [w472 w478] -> w463
          tunnel: [w471 w476] -> w464
          tunnel: w462 -> [w471 w475]
          tunnel: w460 -> [_ w474]
          frame False {
          }
          frame True {
            n185 = property class="Serial Instr"(reference=w484, error in=w483) -> (reference out=w480:refnum<visa-resource-name>, error out=w481:errorcluster, "Serial Settings:Number of Bytes at Serial Port"=w477:u32)
            n186 = Not Equal To 0?(x=w477) -> (x != 0?=w482:bool)
            n187 = case shown="True" w482 {
              tunnel: w481 -> [w487 w495]
              tunnel: w480 -> [w486 w496]
              tunnel: [w487 w490] -> w479
              tunnel: [w486 w494] -> w478
              tunnel: w477 -> [_ w493]
              tunnel: [w485 w492] -> w476
              tunnel: w475 -> [w485 _]
              tunnel: w474 -> [_ w489]
              frame False {
              }
              frame True {
                n188 = VISA Read(VISA resource name=w496, byte count=w493, error in (no error)=w495) -> (VISA resource name out=w494:refnum<visa-resource-name>, read buffer=w492:string, error out=w491:errorcluster)  [unwired: 1 out]
                n189 = call-poly "Enqueue Message.vi"("error in (no error)"=w491, "Message"="Actualizar", "Message Queue"=w489) -> ("error out"=w490:errorcluster)  [unwired: 7 in, 1 out]
              }
            }
          }
        }
        n190 = Bundle By Name(cluster=w466, "Serial.Puerto"=w463, "Serial.Buffer"=w464) -> (w465:T2)
      }
      frame "Actualizar" {
        n191 = Unbundle By Name(w519) -> ("Loop Serial"=w518:refnum<queue>)
        n192 = Unbundle By Name(w528) -> ("Serial.Buffer"=w527:string)
        n193 = Spreadsheet String To Array(delimiter (Tab)=",", format string="%X", spreadsheet string=w527, array type (2D Dbl)=dbl[] []) -> (array=w523:dbl[])
        n194 = call-poly "Enqueue Message.vi"("error in (no error)"=w521, "Message"="Mostrar", "Message Queue"=w518) -> ("error out"=w520:errorcluster)  [unwired: 7 in, 1 out]
        n195 = Index Array(array=w523) -> (element #1=w516:dbl, element #2=w515:dbl, element #3=w514:dbl, element #4=w510:dbl, element #5=w509:dbl, element #6=w508:dbl, element #7=w501:dbl, element #8=w502:dbl, element #9=w503:dbl, element #10=w504:dbl, element #11=w522:dbl)  [unwired: 11 in]
        n196 = call "Hex2Signed.vi"("IN"=w516) -> ("OUT"=w513:dbl)
        n197 = call "Hex2Signed.vi"("IN"=w515) -> ("OUT"=w512:dbl)
        n198 = call "Hex2Signed.vi"("IN"=w514) -> ("OUT"=w511:dbl)
        n199 = To Long Integer(number=w503) -> (32bit integer=w498:i32)
        n200 = To Long Integer(number=w504) -> (32bit integer=w497:i32)
        n201 = To Long Integer(number=w501) -> (32bit integer=w500:i32)
        n202 = To Long Integer(number=w502) -> (32bit integer=w499:i32)
        n203 = call "Hex2Signed.vi"("IN"=w510) -> ("OUT"=w507:dbl)
        n204 = call "Hex2Signed.vi"("IN"=w509) -> ("OUT"=w506:dbl)
        n205 = call "Hex2Signed.vi"("IN"=w508) -> ("OUT"=w505:dbl)
        n206 = Bundle By Name(cluster=w528, "Data.Yaw"=w513, "Data.Pitch"=w512, "Data.Roll"=w511, "Data.Yaw_Desired"=w507, "Data.Pitch_Desired"=w506, "Data.Roll_Desired"=w505, "Data.Motor_Yaw_L"=w500, "Data.Motor_Yaw_R"=w499, "Data.Motor_Pitch_B"=w498, "Data.Motor_Pitch_T"=w497, "Data.Command_Move"=w522) -> (w529:T2)
      }
      frame "Mostrar" {
        n207 = Unbundle By Name(w542) -> ("Data.Yaw"=→"Numeric":dbl, "Data.Pitch"=→"Numeric 2":dbl, "Data.Roll"=→"Numeric 3":dbl, "Data.Yaw_Desired"=→"Numeric 4":dbl, "Data.Pitch_Desired"=→"Numeric 5":dbl, "Data.Roll_Desired"=→"Numeric 6":dbl, "Data.Motor_Yaw_L"=→"Numeric 7":dbl, "Data.Motor_Yaw_R"=→"Numeric 8":dbl, "Data.Motor_Pitch_B"=→"Numeric 9":dbl, "Data.Motor_Pitch_T"=→"Numeric 10":dbl, "Data.Command_Move"=→"Numeric 11":dbl)
      }
    }
    n208 = call "Error Handler - Message Handling Loop.vi"("error in (no error)"=w382, "Message Queue"=w386) -> ("dup error in"=w381:errorcluster)  [unwired: 8 in, 1 out]
  }
  n209 = Unregister For Events(event registration refnum=w11, error in=w9) -> (error out=w12:errorcluster)
  n210 = Merge Errors(w12, w16, w1) -> (w13:errorcluster)
  n211 = call "Destroy User Event - Stop.vi"("error in (no error)"=w13, "User Event - Stop"=w7) -> ("error out"=w10:errorcluster)  [unwired: 9 in]
  n212 = disable-structure shown="Default" {
    disable-tunnel: w10 -> [_ _]
    frame condition #0 (active) {
    }
    frame condition #1 {
      n213 = Quit LabVIEW() -> ()  [unwired: 1 in]
    }
  }
